vi "4.7.vi"() -> ()   [LabVIEW 2017]
panel:
  out "随机数":i32
  out "输入值":i32
  out "猜的次数":i32
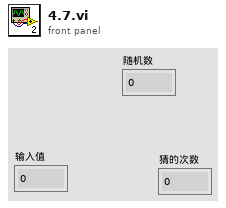
[diagram p1: front panel]
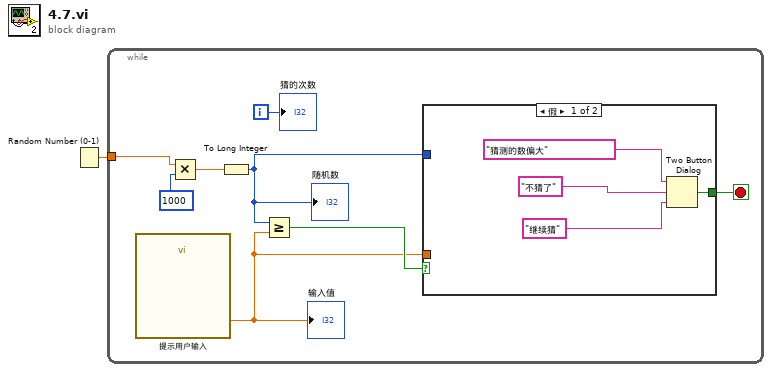
[diagram p0: block diagram]
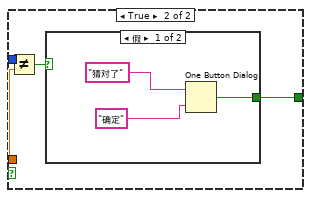
[diagram p2: hidden frame]
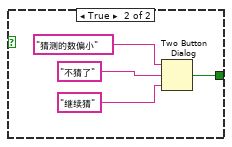
[diagram p3: hidden frame]
diagram:
  n1 = Random Number (0-1)() -> (number: 0 to 1=w1:dbl)
  n2 = while {
    tunnel: w1 -> [w2]
    i -> [w7]
    stop <- w8 stop-if-true
    n3 = call "提示用户输入"() -> ("请在1-1000猜"=w5:dbl)  [unwired: 17 in, 2 out]
    "输入值" <- w5
    n4 = Multiply(x=w2, y=1000) -> (x*y=w4:dbl)
    n5 = To Long Integer(number=w4) -> (32bit integer=w3:i32)
    "随机数" <- w3
    n6 = Greater Or Equal?(x=w3, y=w5) -> (x >= y?=w6:bool)
    n7 = case shown="假" w6 {
      tunnel: w5 -> [_ w14]
      tunnel: w3 -> [_ w15]
      tunnel: [w12 w17] -> w8
      frame False {
        n8 = Two Button Dialog(message="猜测的数偏大", 1:"继续猜", 2:"不猜了") -> (T button?=w12:bool)
      }
      frame True {
        n9 = Not Equal?(x=w15, y=w14) -> (x != y?=w16:bool)
        n10 = case shown="假" w16 {
          tunnel: [w18 w23] -> w17
          frame False {
            n11 = One Button Dialog(message="猜对了", button name ("OK")="确定") -> (true=w18:bool)
          }
          frame True {
            n12 = Two Button Dialog(message="猜测的数偏小", 1:"继续猜", 2:"不猜了") -> (T button?=w23:bool)
          }
        }
      }
    }
    "猜的次数" <- w7
  }
